vi "Obtain Request Events.vi"(8 "error in":errorcluster, 10 "Create New? (F)":bool) -> (0 "error out":errorcluster, 2 "TDMS Request Events":T1)   [LabVIEW 2021, in "TDMS.lvlib"]
doc: "This VI Obtains/Creates the Requests events that will be used for other modules to communicate with the module that owns this VI. These Requests events will be accessed only via Public API methods for this module.\n\n<b>NOTE</b>: The contents of this VI are automatically generated and modified by the <b>Tools > DQMH Consortium > DQMH</b> utilities. Consider using those utilities instead of making your own modifications to this VI.\n_____\nBased on DQMH Project Template 7.0.1.1316."
uses:
  TDMS.lvlib
  Request Events--cluster.ctl
  Stop Argument--cluster.ctl
  Show Panel Argument--cluster.ctl
  Hide Panel Argument--cluster.ctl
  Get Module Execution Status Argument--cluster.ctl
  Show Diagram Argument--cluster.ctl
  Create TDMS File Argument--cluster.ctl
  Close TDMS File Argument--cluster.ctl
  Write Data Argument--cluster.ctl
  RT Main/Data Cluster.ctl
  Libraries/Common RT/Hardware Monitoring.ctl
  Write Data to File Argument--cluster.ctl
  RT Main/RT Main.lvlib
  Libraries/Common RT/Common RT.lvlib
panel:
  # "NOTE: The contents of this VI are automatically generated and modified by the Tools > DQMH Consortium > DQMH utilities. Consider using those utilities instead of making your own modifications to this VI."
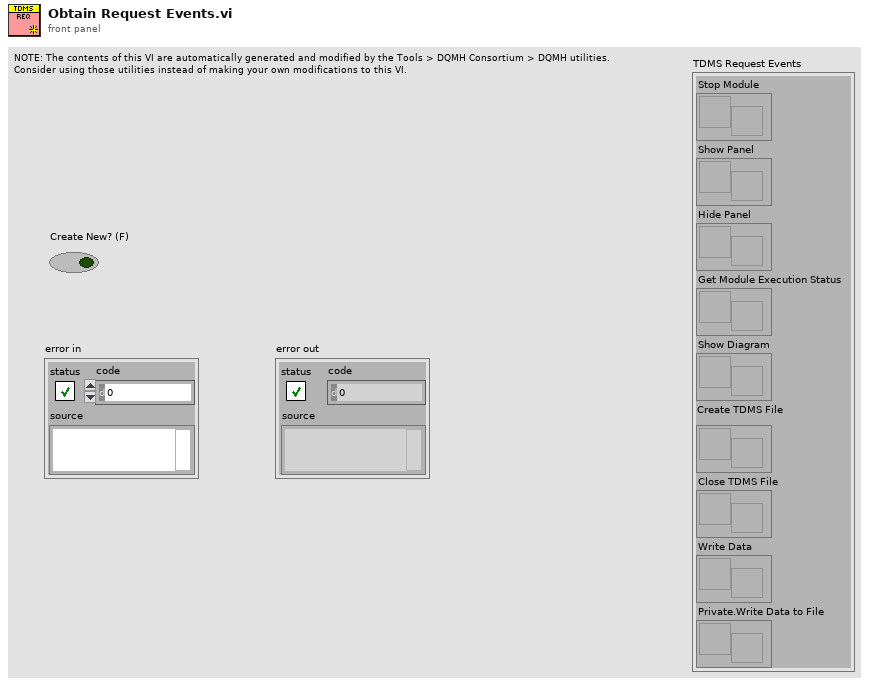
[diagram p1: front panel]
types:
  T1 = typedef "TDMS.lvlib/Request Events--cluster.ctl" = cluster{"Stop Module":refnum<user-event>, "Show Panel":refnum<user-event>, "Hide Panel":refnum<user-event>, "Get Module Execution Status":refnum<user-event>, "Show Diagram":refnum<user-event>, "Create TDMS File":refnum<user-event>, "Close TDMS File":refnum<user-event>, "Write Data":refnum<user-event>, "Private.Write Data to File":refnum<user-event>}
  T2 = typedef "TDMS.lvlib/Write Data to File Argument--cluster.ctl" = cluster{"Data Cluster":T3[]}
  T3 = typedef "RT Main.lvlib/Data Cluster.ctl" = cluster{"Analog Input":dbl[], "Digital Inputs":bool[], "System Status":T4, "Iteration Duration (ms)":dbl, "Finish Late?":bool}
  T4 = typedef "Common RT.lvlib/Hardware Monitoring.ctl" = cluster{"Memory RAM Free (%)":dbl, "Free Flash memory (%)":dbl, "CPU 0 (%)":u32, "CPU 1 (%)":u32}
  T5 = typedef "TDMS.lvlib/Write Data Argument--cluster.ctl" = cluster{"Data":T3[]}
  T6 = typedef "TDMS.lvlib/Close TDMS File Argument--cluster.ctl" = cluster{"Boolean":bool}
  T7 = typedef "TDMS.lvlib/Create TDMS File Argument--cluster.ctl" = cluster{"Boolean":bool}
  T8 = typedef "TDMS.lvlib/Hide Panel Argument--cluster.ctl" = cluster{"Hide Panel?":bool}
  T9 = typedef "TDMS.lvlib/Show Panel Argument--cluster.ctl" = cluster{"Show Panel?":bool}
  T10 = typedef "TDMS.lvlib/Show Diagram Argument--cluster.ctl" = cluster{"Debug?":bool}
  T11 = typedef "TDMS.lvlib/Get Module Execution Status Argument--cluster.ctl" = cluster{"Running?":bool}
  T12 = typedef "TDMS.lvlib/Stop Argument--cluster.ctl" = cluster{"Origin":string, "Exit via Stop Module Req?":bool, "Wait for Module to stop?":bool}
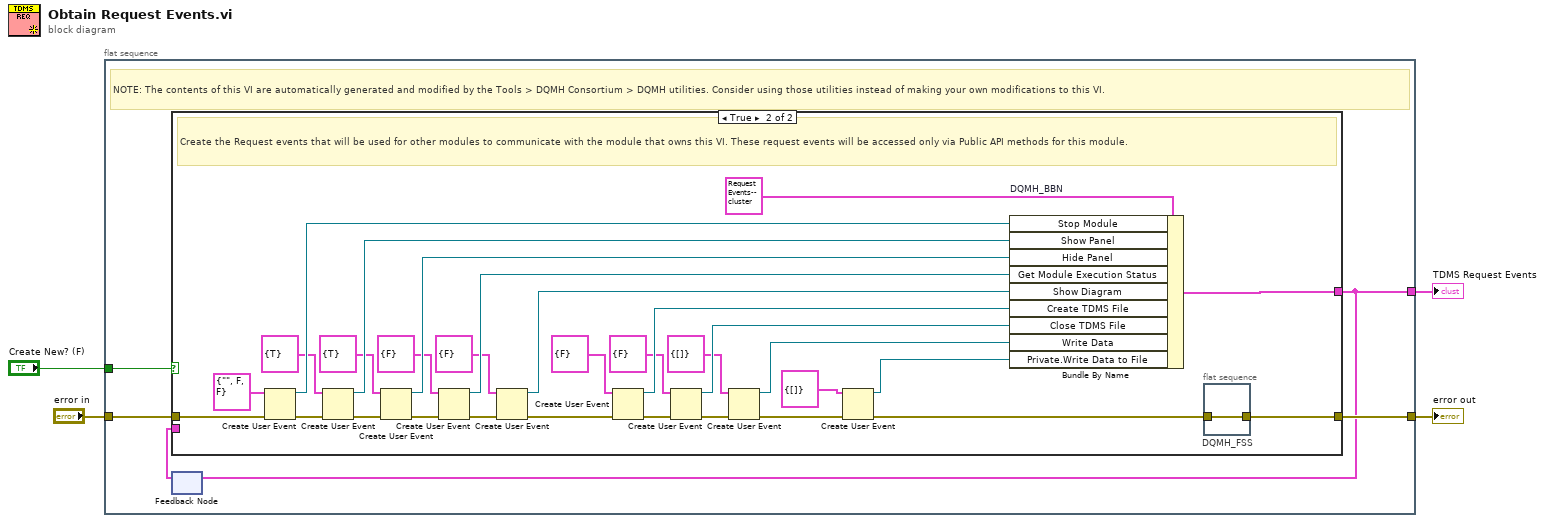
[diagram p0: block diagram]
diagram:
  n1 = flat-sequence {
    tunnel: [w9] -> w4
    tunnel: "error in" -> [w8]
    tunnel: [w6] -> w2
    tunnel: "Create New? (F)" -> [w5]
    frame #0 {
      # "NOTE: The contents of this VI are automatically generated and modified by the Tools > DQMH Consortium > DQMH utilities. Consider using those utilities instead of making your own modifications to this VI."
      n2 = feedback #1() -> (w7:T1)  [unwired: 1 in]
      n3 = case shown="True" w5 {
        tunnel: [w10 w32] -> w9
        tunnel: w8 -> [w10 w42]
        tunnel: [w11 w39] -> w6
        tunnel: w7 -> [w11 _]
        frame False {
          # "Obtain the Request events that were created in a previous call to this VI."
        }
        frame True {
          # "Create the Request events that will be used for other modules to communicate with the module that owns this VI. These request events will be accessed only via Public API methods for this module."
          n4 = Create User Event(user event datatype=T12 {"Origin"="", "Exit via Stop Module Req?"=FALSE, "Wait for Module to stop?"=FALSE} ("Stop Argument"), error in=w42) -> (user event=w40:refnum<user-event>, error out=w37:errorcluster)
          n5 = Create User Event(user event datatype=T9 {"Show Panel?"=TRUE} ("Show Panel Argument"), error in=w37) -> (user event=w36:refnum<user-event>, error out=w35:errorcluster)
          n6 = Create User Event(user event datatype=T8 {"Hide Panel?"=TRUE} ("Hide Panel Argument"), error in=w35) -> (user event=w34:refnum<user-event>, error out=w33:errorcluster)
          n7 = Create User Event(user event datatype=T11 {"Running?"=FALSE} ("Get Module Execution Status Argument"), error in=w33) -> (user event=w30:refnum<user-event>, error out=w31:errorcluster)
          n8 = Create User Event(user event datatype=T10 {"Debug?"=FALSE} ("Show Diagram Argument"), error in=w31) -> (user event=w27:refnum<user-event>, error out=w28:errorcluster)
          n9 = Create User Event(user event datatype=T7 {"Boolean"=FALSE} ("Create TDMS File Argument"), error in=w28) -> (user event=w23:refnum<user-event>, error out=w21:errorcluster)
          n10 = Create User Event(user event datatype=T6 {"Boolean"=FALSE} ("Close TDMS File Argument"), error in=w21) -> (user event=w18:refnum<user-event>, error out=w20:errorcluster)
          n11 = Create User Event(user event datatype=T5 {"Data"=[]} ("Write Data Argument"), error in=w20) -> (user event=w17:refnum<user-event>, error out=w13:errorcluster)
          n12 = Create User Event(user event datatype=T2 {"Data Cluster"=[]} ("Write Data to File Argument"), error in=w13) -> (user event=w14:refnum<user-event>, error out=w12:errorcluster)
          n13 = Bundle By Name "DQMH_BBN"(cluster=T1 {"Stop Module"=refnum, "Show Panel"=refnum, "Hide Panel"=refnum, "Get Module Execution Status"=refnum, "Show Diagram"=refnum, "Create TDMS File"=refnum, "Close TDMS File"=refnum, "Write Data"=refnum, "Private.Write Data to File"=refnum} ("output cluster"), "Stop Module"=w40, "Show Panel"=w36, "Hide Panel"=w34, "Get Module Execution Status"=w30, "Show Diagram"=w27, "Create TDMS File"=w23, "Close TDMS File"=w18, "Write Data"=w17, "Private.Write Data to File"=w14) -> (w39:T1)
          n14 = flat-sequence "DQMH_FSS" {
            tunnel: w12 -> [w43]
            tunnel: [w43] -> w32
            frame #0 {
            }
          }
        }
      }
      n15 = feedback-in #1(w6) -> ()
    }
  }
  "TDMS Request Events" <- w2
  "error out" <- w4
